vi "Animated GIF Example.vi"() -> ()   [LabVIEW 2020]
doc: "G-Image example demonstrating image loading, rotation, and display."
uses:
  Image IO/Polymorphic VIs/Load Animated GIF Image (Path).vi
  G-Image.lvlib
panel:
  in  "Playback Speed":dbl(slide)=1.0 min=0.25 max=5.0 step=0.25 scale=0.25..5.0
  in  "Stop":bool
  out "2D Picture":picture
  # "Instructions:\n1. Run the VI.\n2. Adjust the playback speed using the slider."
  # "G"
  # "-Image"
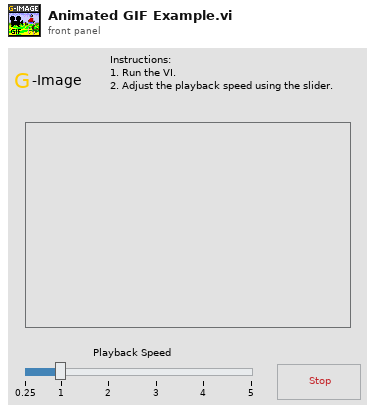
[diagram p1: front panel]
types:
  T1 = typedef "imagedata.ctl" = cluster{"image type":i32, "image depth":i32, "image":u8[], "mask":u8[], "colors":u32[], "Rectangle":cluster{"left":i16, "top":i16, "right":i16, "bottom":i16}}
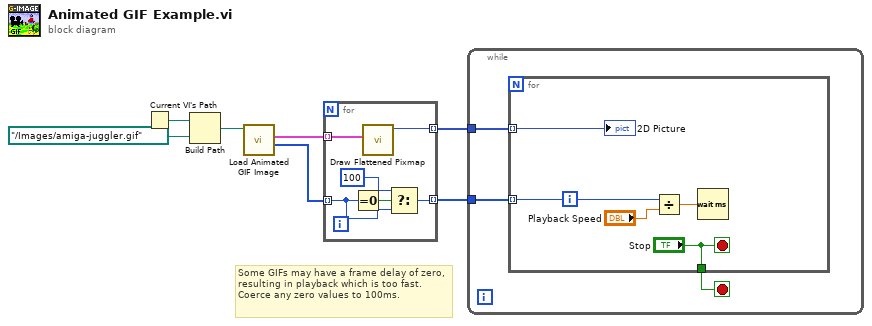
[diagram p0: block diagram]
diagram:
  # "Some GIFs may have a frame delay of zero, resulting in playback which is too fast. Coerce any zero values to 100ms."
  n1 = Current VI's Path() -> (path=w7:path)
  n2 = Build Path(base path=w7, name or relative path=path "../Images/amiga-juggler.gif") -> (appended path=w5:path)
  n3 = call-poly "Load Animated GIF Image.vi"("Path In"=w5) -> ("Delays"=w4:i32[], "Frames"=w2:T1[])  [unwired: 7 in, 2 out]
  n4 = for {
    tunnel: w4 -> [w11] mode=indexing
    tunnel: [w10] -> w3 mode=indexing
    tunnel: w2 -> [w9] mode=indexing
    tunnel: [w8] -> w1 mode=indexing
    n5 = Equal To 0?(x=w11) -> (x = 0?=w13:bool)
    n6 = call <vilib>:"Draw Flattened Pixmap.vi"("image data"=w9) -> ("new picture"=w8:picture)  [unwired: 8 in]
    n7 = Select(t=100, s=w13, f=w11) -> (s? t:f=w10:i32)
  }
  n8 = while {
    tunnel: w1 -> [w16]
    tunnel: w3 -> [w15]
    stop <- w14 stop-if-true
    n9 = for {
      tunnel: w16 -> [w17] mode=indexing
      tunnel: w15 -> [w19] mode=indexing
      tunnel: ["Stop"] -> w14
      stop <- "Stop" stop-if-true
      n10 = Divide(x=w19, y="Playback Speed") -> (x/y=w18:dbl)
      n11 = Wait (ms)(milliseconds to wait=w18) -> ()  [unwired: 1 out]
      "2D Picture" <- w17
    }
  }
